vi "Read Cluster Size.vi"(9 "Cluster in":refnum<class "Cluster.lvclass">) -> (3 "Cluster out":refnum<class "Cluster.lvclass">, 4 "Cluster Size":T1)   [LabVIEW 2014, in "Cluster.lvclass"]
uses:
  Cluster.lvclass
  <vilib>/Utility/miscctls.llb/LVBoundsTypeDef.ctl
  Cluster.lvclass/Cluster.ctl
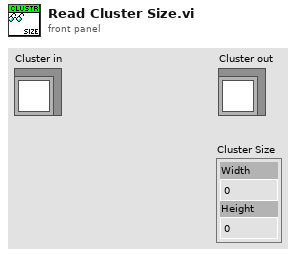
[diagram p1: front panel]
types:
  T1 = typedef "LVBoundsTypeDef.ctl" = cluster{"Width":u32, "Height":u32}
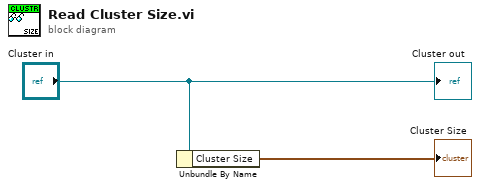
[diagram p0: block diagram]
diagram:
  n1 = Unbundle By Name("Cluster in") -> ("Cluster Size"=→"Cluster Size":T1)
  "Cluster out" <- "Cluster in"
